vi "Destroy.vi"(0 "reference in":refnum<class "IMyInterface.lvclass">, 5 "error in (no error)":errorcluster) -> (14 "reference out":refnum<class "IMyInterface.lvclass">, 19 "error out":errorcluster)   [LabVIEW 2020, in "IMyInterface.lvclass"]
doc: "Destructor."
uses:
  IMyInterface.lvclass
  vi.lib/addons/_AddQ/G#Interface/G#Interface.lvclass
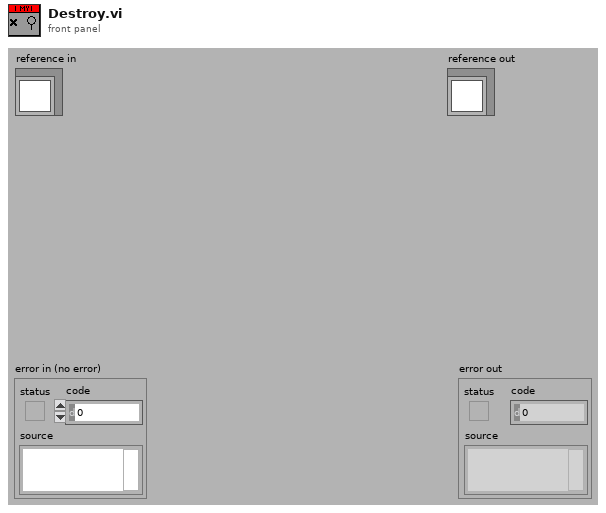
[diagram p1: front panel]
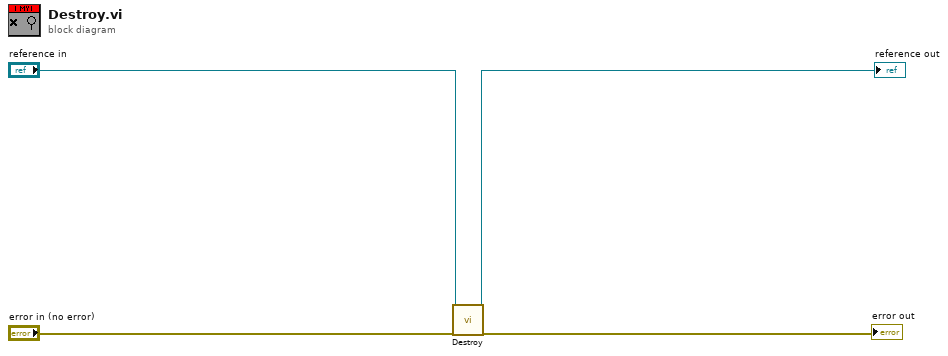
[diagram p0: block diagram]
diagram:
  n1 = call-parent "Destroy.vi"("reference in"="reference in", "error in (no error)"="error in (no error)") -> ("reference out"=→"reference out":refnum<class "IMyInterface.lvclass">, "error out"=→"error out":errorcluster)  [unwired: 16 in]
